vi "FdxCmdRxSAPBlockReadCvi.vi"(8 "error in":errorcluster, 9 "SapBlockReadIn":T2, 11 "InstrumentHandle_port":u32) -> (0 "error out":errorcluster, 1 "SapBlockReadOut":T1, 3 "InstrumentHandle_port":u32)   [LabVIEW 2020, in "AIM664LV.lvlib"]
doc: "This function reads data from one or several SAP connectionless ports."
uses:
  AIM664LV.lvlib
  AFDX_LibraryAdmin/FdxGlobalDllPath.vi
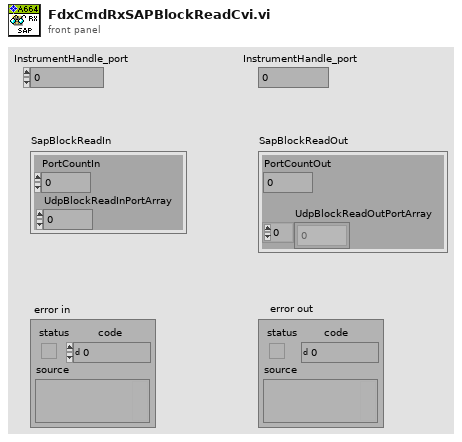
[diagram p1: front panel]
types:
  T1 = cluster{"PortCountOut":u32, "UdpBlockReadOutPortArray":u8[]}
  T2 = cluster{"PortCountIn":u32, "UdpBlockReadInPortArray":u32}
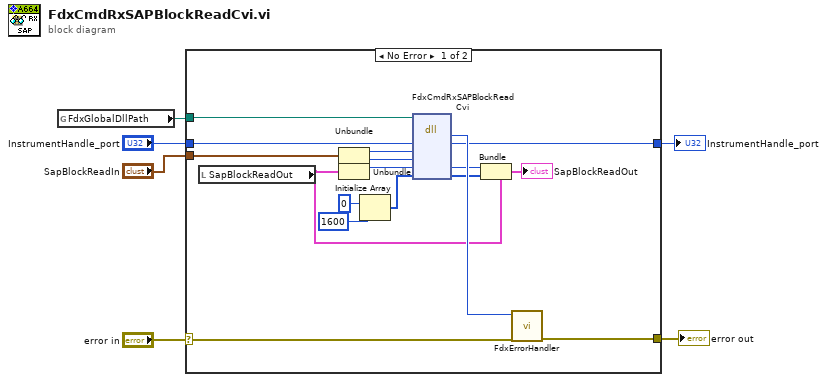
[diagram p0: block diagram]
diagram:
  n1 = global read "FdxGlobalDllPath.vi" "FdxGlobalDllPath"() -> (w4:path)
  n2 = case shown="No Error" "error in" {
    selector: "error in" -> [w22 w25]
    tunnel: [w23 w25] -> w6
    tunnel: w4 -> [w10 _]
    tunnel: "InstrumentHandle_port" -> [w9 w24]
    tunnel: [w8 w24] -> w2
    tunnel: "SapBlockReadIn" -> [w7 _]
    frame No Error {
      n3 = local read "SapBlockReadOut"() -> (w12:T1)
      n4 = Unbundle(w7) -> ("PortCountIn"=w19:u32, "UdpBlockReadInPortArray"=w18:u32)
      n5 = Unbundle(w12) -> ("PortCountOut"=w11:u32)  [unwired: 1 out]
      n6 = Initialize Array(u8 0 ("element"), 1600 ("dimension size")) -> (w14:u8[])
      n7 = dll-call lib="aim_fdx.19.dll" fn="FdxCmdRxSAPBlockReadCvi"(path in=w10, "InstrumentHandle"=w9, "PortCountIn"=w19, "UdpBlockReadInPortArray"=w18, "PortCountOut"=w11, "UdpBlockReadOutPortArray"=w14) -> ("status"=w21:i32, "InstrumentHandle"=w8:u32, "PortCountOut"=w17:u32, "UdpBlockReadOutPortArray"=w13:u8[])  [unwired: 3 in, 3 out]
      n8 = Bundle(cluster=w12, "PortCountOut"=w17, "UdpBlockReadOutPortArray"=w13) -> (→"SapBlockReadOut":T1)
      n9 = call "FdxErrorHandler.vi"("error in"=w22, "AIM Error"=w21) -> ("error out"=w23:errorcluster)  [unwired: 9 in]
    }
    frame Error {
    }
  }
  "error out" <- w6
  "InstrumentHandle_port" <- w2
